vi "LVClass_HasoData Set Compute Phase Set.vi"(0 "HasoData in":refnum<class "HasoData.lvclass">, 5 "ComputePhaseSet in":refnum<class "ComputePhaseSet.lvclass">, 7 "ModalCoef in":refnum<class "ModalCoef.lvclass">, 11 "error in (no error)":errorcluster) -> (4 "HasoData out":refnum<class "HasoData.lvclass">, 6 "ComputePhaseSet out":refnum<class "ComputePhaseSet.lvclass">, 8 "ModalCoef out":refnum<class "ModalCoef.lvclass">, 15 "error out":errorcluster)   [LabVIEW 2020, in "HasoData.lvclass"]
doc: "Set ComputePhaseSet object.\n\n--------------------------------------------------------------------------------\n\n<B>HasoDataIn </B> : HasoData object.\n<B>HasoDataOut </B> : HasoData object.\n<B>ComputePhaseSet </B> : ComputePhaseSet object.\n<B>ErrorIn </B> : Error\n<B>ErrorOut </B> : Error\n\n--------------------------------------------------------------------------------"
uses:
  HasoData.lvclass
  ComputePhaseSet/ComputePhaseSet.lvclass
  ModalCoef/ModalCoef.lvclass
  HasoData.lvclass/HasoData.ctl
  ModalCoef/LVClass_ModalCoef Read ModalCoef.vi
  ComputePhaseSet/LVClass_ComputePhaseSet Read ComputePhaseSet.vi
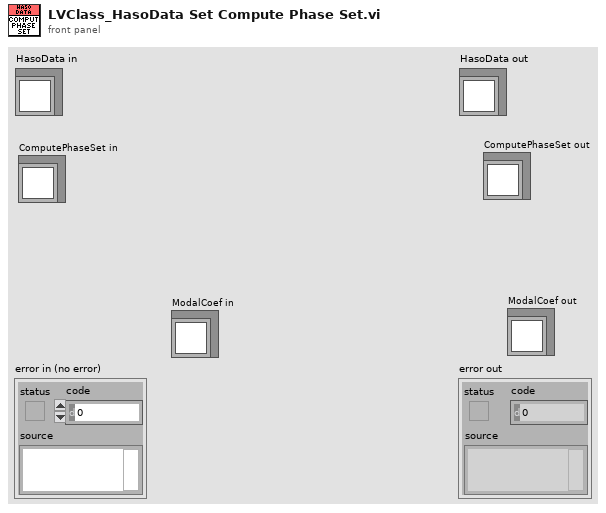
[diagram p1: front panel]
types:
  T1 = typedef "WavefrontReconstructionMode.ctl" = enum16{"None", "Modal_Legendre", "Modal_Zernike", "Zonal", "Modal_Zonal_Zernike", "Modal_Zonal_Legendre"}
  T2 = typedef "ClassID.ctl" = i64
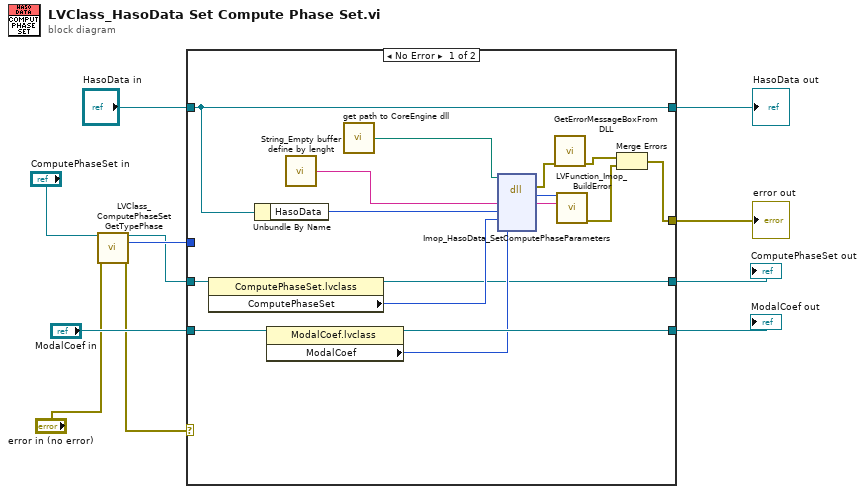
[diagram p0: block diagram]
diagram:
  n1 = call "LVClass_ComputePhaseSet GetTypePhase.vi"("ComputePhaseSet in"="ComputePhaseSet in", "error in (no error)"="error in (no error)") -> ("ComputePhaseSet out"=w3:refnum<class "ComputePhaseSet.lvclass">, "Reconstruction Mode"=w5:T1, "error out"=w1:errorcluster)  [unwired: 11 in]
  n2 = case shown="No Error" w1 {
    selector: w1 -> [_ w31]
    tunnel: [w16 w31] -> w10
    tunnel: [w20 w30] -> w9
    tunnel: "HasoData in" -> [w20 w30]
    tunnel: w3 -> [w22 w28]
    tunnel: "ModalCoef in" -> [w15 w29]
    tunnel: [w14 w29] -> w7
    tunnel: [w12 w28] -> w6
    tunnel: w5 -> [_ _]
    frame No Error {
      n3 = property class="ComputePhaseSet.lvclass"(reference=w22) -> (reference out=w12:refnum<class "ComputePhaseSet.lvclass">, "ComputePhaseSet"=w21:T2)  [unwired: 1 in, 1 out]
      n4 = Unbundle By Name(w20) -> ("HasoData"=w19:T2)
      n5 = property class="ModalCoef.lvclass"(reference=w15) -> (reference out=w14:refnum<class "ModalCoef.lvclass">, "ModalCoef"=w13:T2)  [unwired: 1 in, 1 out]
      n6 = call "String_Empty buffer define by lenght.vi"() -> ("Empty buffer"=w25:string)  [unwired: 1 in]
      n7 = call "get path to CoreEngine dll.vi"() -> ("path to wavekit library"=w24:path)  [unwired: 14 in, 1 out]
      n8 = dll-call lib="D:/2_trunk/Soft_haso/ImOpCoreEngine4_LV2011/DLLs/ImopEngine4_vc100.dll" fn="Imop_HasoData_SetComputePhaseParameters"(path in=w24, "message"=w25, "objet"=w19, "ComputePhaseSet"=w21, "arg5"=w13) -> (error out=w23:errorcluster, "return type"=w27:i32, "message"=w26:string)  [unwired: 5 in, 1 out]
      n9 = call "GetErrorMessageBoxFromDLL.vi"("error IN"=w23) -> ("error OUT"=w18:errorcluster)  [unwired: 10 in]
      n10 = call "LVFunction_Imop_BuildError.vi"("code"=w27, "String to Prepend to source (\"\")"=w26) -> ("error out"=w17:errorcluster)  [unwired: 13 in]
      n11 = Merge Errors(w18, w17) -> (w16:errorcluster)
    }
    frame Error {
    }
  }
  "error out" <- w10
  "HasoData out" <- w9
  "ModalCoef out" <- w7
  "ComputePhaseSet out" <- w6
